vi "arrayfunctions.vi"() -> ()   [LabVIEW 2015]
panel:
  in  "Tab Control":T1(tab)
  out "Size of the array":i32
  in  "index":i32
  out "element":dbl
  out "Resultado":dbl[](array[numeric]) format="%#.2f"
  in  "Indexes":i16[](array[numeric])
  in  "Elements":dbl[](array[numeric])
  in  "Index para agregar":i32
  out "Resultado":dbl[](array[numeric]) format="%#.2f"
  in  "length":i32
  in  "First element":i32
  out "array w/ subset deleted":dbl[](array[numeric]) format="%#.2f"
  out "deleted portion":dbl[](array[numeric]) format="%#.2f"
  out "Result":dbl[](array[numeric])
  in  "Segundo array":dbl[](array[numeric])
  in  "Primer array":dbl[](array[numeric])
  out "max value":dbl
  out "max index(es)":i32
  out "min value":dbl
  out "min index(es)":i32
  in  "First Shape Indicator":i16
  in  "Second Shape Indicator":i32
  out "output array":dbl[][](array[numeric])
  out "sorted array":dbl[](array[numeric]) format="%#.2f"
  in  "Starting index":i16
  in  "Element that you\n are looking for":dbl
  out "index of element":i32
  in  "Split index":i32
  out "second subarray":dbl[](array[numeric])
  out "first subarray":dbl[](array[numeric])
  out "reversed array":dbl[](array[numeric]) format="%#.2f"
  in  "Number of rotations":i32
  out "array (last n elements first)":dbl[](array[numeric]) format="%#.2f"
  out "Array":dbl[](array[numeric]) format="%#.2f"
  in  "stop":bool
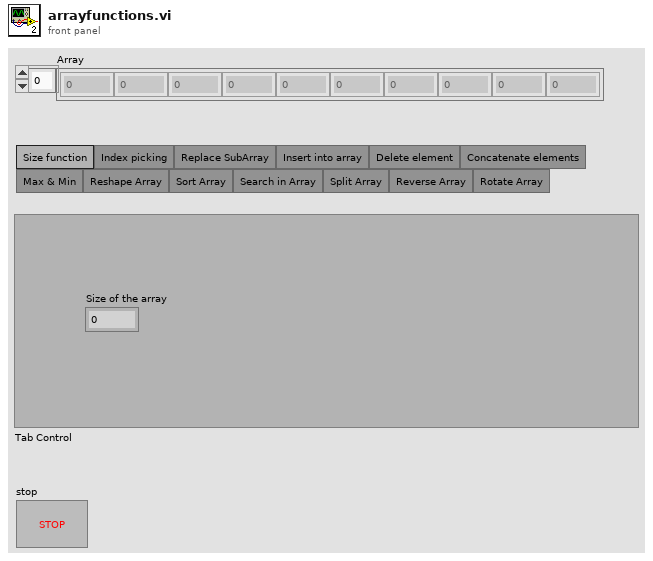
[diagram p1: front panel]
types:
  T1 = enum32{"Size function", "Index picking", "Replace SubArray", "Insert into array", "Delete element", "Concatenate elements", "Max & Min", "Reshape Array", "Sort Array", "Search in Array", "Split Array", "Reverse Array", "Rotate Array"}
  T2 = cluster{"Indexes[0]":i16, "Indexes[1]":i16, "Indexes[2]":i16, "Indexes[3]":i16, "Indexes[4]":i16, "Indexes[5]":i16, "Indexes[6]":i16, "Indexes[7]":i16, "Indexes[8]":i16}
  T3 = cluster{"Elements[0]":dbl, "Elements[1]":dbl, "Elements[2]":dbl, "Elements[3]":dbl, "Elements[4]":dbl, "Elements[5]":dbl, "Elements[6]":dbl, "Elements[7]":dbl, "Elements[8]":dbl}
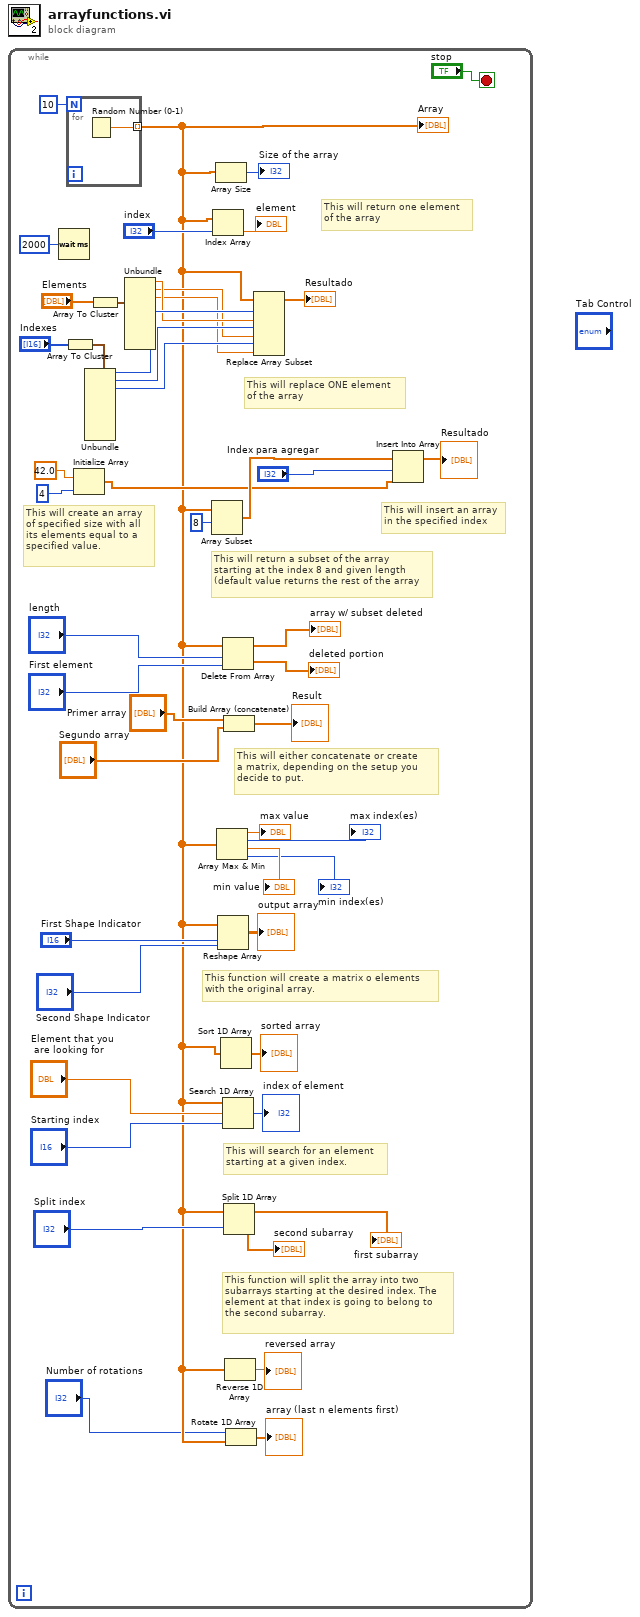
[diagram p0: block diagram]
diagram:
  n1 = while {
    stop <- "stop" stop-if-true
    # "This function will split the array into two \nsubarrays starting at the desired index. The\nelement at that index is going to belong to \nthe second subarray."
    # "This will search for an element\nstarting at a given index."
    # "This function will create a matrix o elements\nwith the original array."
    # "This will either concatenate or create\na matrix, depending on the setup you \ndecide to put."
    # "This will create an array\nof specified size with all \nits elements equal to a \nspecified value."
    # "This will insert an array\nin the specified index"
    # "This will return a subset of the array\nstarting at the index 8 and given length\n(default value returns the rest of the array"
    # "This will return one element\nof the array"
    # "This will replace ONE element\nof the array"
    n2 = Wait (ms)(milliseconds to wait=u32 2000) -> ()  [unwired: 1 out]
    n3 = Array To Cluster(array="Indexes") -> (cluster=w43:T2)
    n4 = for {
      N: 10 -> [_]
      tunnel: [w50] -> w3 mode=indexing
      n5 = Random Number (0-1)() -> (number: 0 to 1=w50:dbl)
    }
    "Array" <- w3
    n6 = Initialize Array(42.0 ("element"), 4 ("dimension size")) -> (w27:dbl[])
    n7 = Unbundle(w43) -> ("Indexes[0]"=w42:i16, "Indexes[1]"=w41:i16, "Indexes[2]"=w40:i16)  [unwired: 6 out]
    n8 = Array To Cluster(array="Elements") -> (cluster=w38:T3)
    n9 = Unbundle(w38) -> ("Elements[0]"=w36:dbl, "Elements[1]"=w35:dbl, "Elements[2]"=w34:dbl)  [unwired: 6 out]
    n10 = Array Subset(array=w3, index=8) -> (w31:dbl[])  [unwired: 1 in]
    n11 = Index Array(array=w3, index="index") -> (element=→"element":dbl)
    n12 = Array Size(array=w3) -> (size(s)=→"Size of the array":i32)
    n13 = Array Max & Min(array=w3) -> (max value=→"max value":dbl, max index (indices)=→"max index(es)":i32, min value=→"min value":dbl, min index (indices)=→"min index(es)":i32)
    n14 = Reshape Array(w3, "First Shape Indicator", "Second Shape Indicator") -> (→"output array":dbl[][])
    n15 = Sort 1D Array(array=w3) -> (sorted array=→"sorted array":dbl[])
    n16 = Delete From Array(array=w3, length="length", index="First element") -> (deleted portion=→"deleted portion":dbl[], array with subset deleted=→"array w/ subset deleted":dbl[])
    n17 = Search 1D Array(1D array=w3, element="Element that you\n are looking for", start index (0)="Starting index") -> (index of element=→"index of element":i32)
    n18 = Build Array (concatenate)("Primer array", "Segundo array") -> (→"Result":dbl[])
    n19 = Split 1D Array(array=w3, index="Split index") -> (first subarray=→"first subarray":dbl[], second subarray=→"second subarray":dbl[])
    n20 = Reverse 1D Array(array=w3) -> (reversed array=→"reversed array":dbl[])
    n21 = Rotate 1D Array(1:w3, 2:"Number of rotations") -> (0:→"array (last n elements first)":dbl[])
    n22 = Replace Array Subset(array=w3, new element #1=w36, index #1=w42, new element #2=w35, index #2=w41, new element #3=w34, index #3=w40) -> (→"Resultado":dbl[])
    n23 = Insert Into Array(array=w31, index="Index para agregar", new element=w27) -> (→"Resultado":dbl[])
  }
